vi "test.vi"() -> ()   [LabVIEW 2025]
panel:
  in  "Number of trials":dbl=1.0 min=1.0 step=1.0
  out "Final Door Probability":dbl
  out "Win Rate Stay":dbl
  out "Win Rate Switch":dbl
  in  "Number of Doors":dbl=3.0 min=3.0 step=1.0
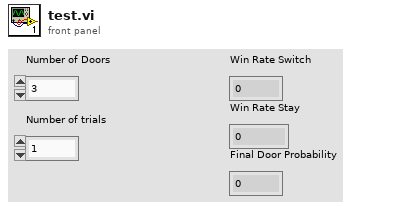
[diagram p1: front panel]
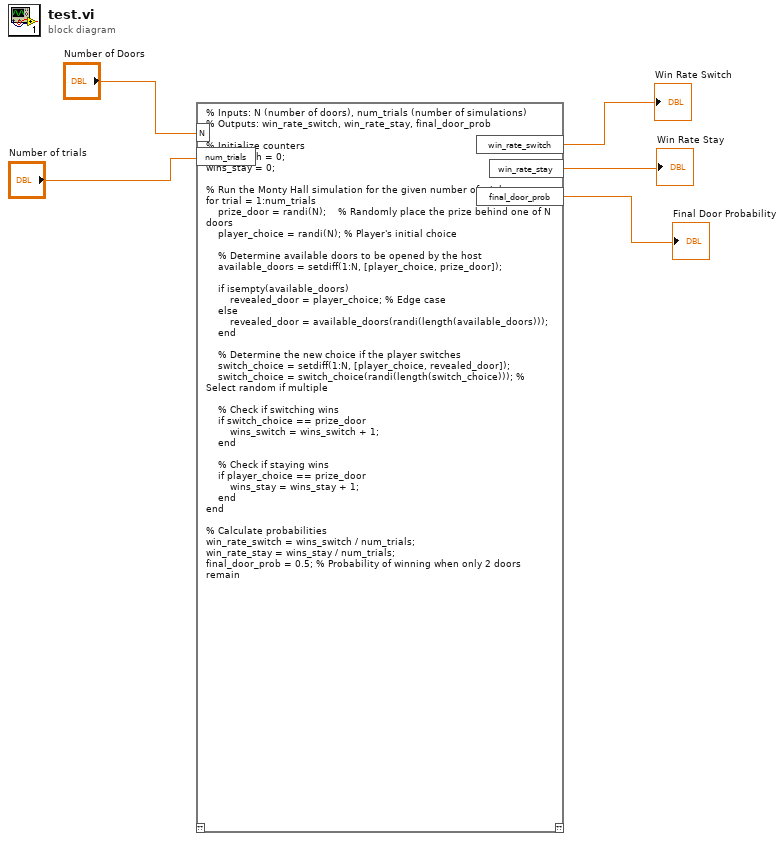
[diagram p0: block diagram]
diagram:
  n1 = script code="% Inputs: N (number of doors), num_trials (number of simulations)\n% Outputs: win_rate_switch, win_rate_stay, final_door_prob\n\n% Initialize counters\nwins_switch = 0;\nwins_stay = 0;\n\n% Run the Monty Hall simulation for the given number of trials\nfor trial = 1:num_trials\n    prize_door = randi(N);    % Randomly place the prize behind one of N doors\n    player_choice = randi(N); % Player's initial choice\n\n    % Determine available doors to be opened by the host\n    available_doors = setdiff(1:N, [player_choice, prize_door]);\n    \n    if isempty(available_doors)\n        revealed_door = player_choice; % Edge case\n    else\n        revealed_door = available_doors(randi(length(available_doors)));\n    end\n    \n    % Determine the new choice if the player switches\n    switch_choice = setdiff(1:N, [player_choice, revealed_door]);\n    switch_choice = switch_choice(randi(length(switch_choice))); % Select random if multiple\n    \n    % Check if switching wins\n    if switch_choice == prize_door\n        wins_switch = wins_switch + 1;\n    end\n    \n    % Check if staying wins\n    if player_choice == prize_door\n        wins_stay = wins_stay + 1;\n    end\nend\n\n% Calculate probabilities\nwin_rate_switch = wins_switch / num_trials;\nwin_rate_stay = wins_stay / num_trials;\nfinal_door_prob = 0.5; % Probability of winning when only 2 doors remain"("N"="Number of Doors", "num_trials"="Number of trials") -> ("win_rate_switch"=→"Win Rate Switch":dbl, "win_rate_stay"=→"Win Rate Stay":dbl, "final_door_prob"=→"Final Door Probability":dbl)  [unwired: 1 in, 1 out]
